vi "Err.vi"(6 "source":string="CreateDevice Error.", 8 "error in (no error)":errorcluster, 9 "Par":i32[](array[numeric]), 10 "error?":bool, 11 "code":i32) -> (0 "error out":errorcluster)   [LabVIEW 2009]
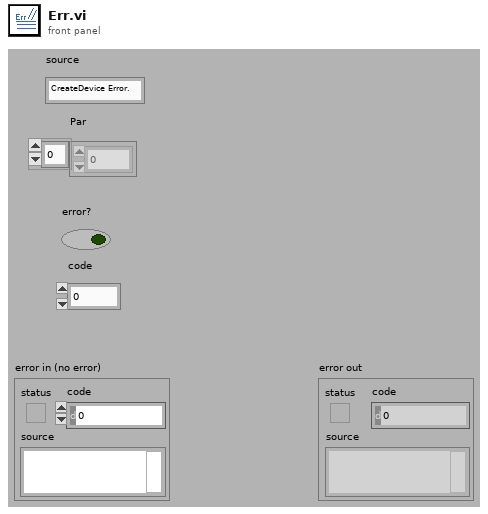
[diagram p1: front panel]
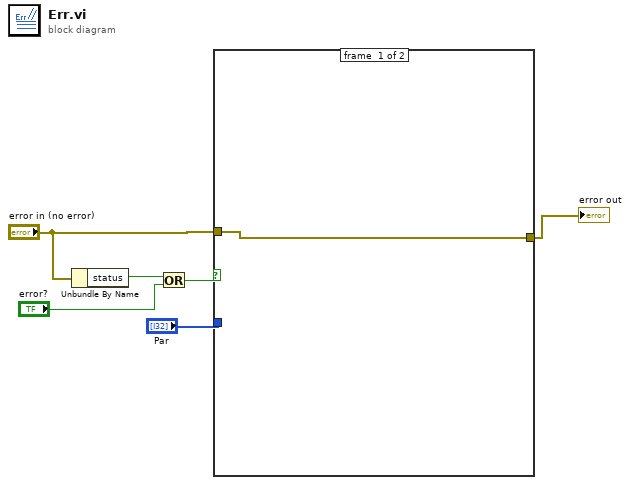
[diagram p0: block diagram]
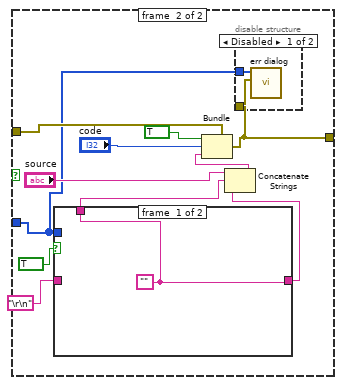
[diagram p2: hidden frame]
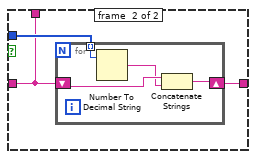
[diagram p4: hidden frame]
diagram:
  n1 = Unbundle By Name("error in (no error)") -> ("status"=w3:bool)
  n2 = Or(x=w3, y="error?") -> (x .or. y?=w4:bool)
  n3 = case shown="真" w4 {
    tunnel: "error in (no error)" -> [w7 w17]
    tunnel: [w7 w9] -> w5
    tunnel: "Par" -> [_ w8]
    frame #0 {
    }
    frame #1 {
      n4 = case shown="真" TRUE {
        tunnel: w8 -> [_ w24]
        tunnel: "\r\n" -> [_ w22]
        tunnel: [w21 w23] -> w13
        tunnel: [w21 w22] -> w12
        frame #0 {
          w21 = ""
        }
        frame #1 {
          n5 = for {
            tunnel: w24 -> [w28] mode=indexing
            shift-right: [w25] -> w23
            shift-left: w22 -> [w27]
            n6 = Number To Decimal String(number=w28) -> (decimal integer string=w26:string)  [unwired: 1 out]
            n7 = Concatenate Strings(w27, w26) -> (w25:string)
          }
        }
      }
      n8 = Concatenate Strings("source", w12, w13) -> (w10:string)
      n9 = Bundle(cluster=w17, "status"=TRUE, "code"="code", "source"=w10) -> (w9:errorcluster)
      n10 = disable-structure shown="Disabled" {
        disable-tunnel: w9 -> [w20 _]
        disable-tunnel: w8 -> [w19 _]
        frame #0 {
          n11 = call "err dialog.vi"("错误提示 2"=w20, "参数 2"=w19) -> ()  [unwired: 10 out]
        }
        frame #1 {
        }
      }
    }
  }
  "error out" <- w5
